vi "test-AprilTag-Test2.vi"() -> (3 "All Passed":bool)   [LabVIEW 2019]
uses:
  <vilib>/Rock Robotics/WPI/ThirdParty/JAS_Junk/TrajLib/TypeDef/AprilTagFieldLayout.ctl
  <vilib>/Rock Robotics/WPI/ThirdParty/JAS_Junk/TrajLib/TypeDef/AprilTag.ctl
  <vilib>/Rock Robotics/WPI/ThirdParty/JAS_Junk/TrajLib/TypeDef/POSE3D.ctl
  <vilib>/Rock Robotics/WPI/ThirdParty/JAS_Junk/TrajLib/TypeDef/TRANSLATION3D.ctl
  <vilib>/Rock Robotics/WPI/ThirdParty/JAS_Junk/TrajLib/TypeDef/ROTATION3D.ctl
  <vilib>/Rock Robotics/WPI/ThirdParty/JAS_Junk/TrajLib/TypeDef/QUATERNION.ctl
  <vilib>/Rock Robotics/WPI/ThirdParty/JAS_Junk/TrajLib/Enum/AprilTagFieldLayoutOrignPosition_ENUM.ctl
  <vilib>/Rock Robotics/WPI/ThirdParty/JAS_Junk/TrajLib/Conv_Deg_Radians.vi
  <vilib>/Rock Robotics/WPI/ThirdParty/JAS_Junk/TrajLib/VI/Quaternion_New.vi
  <vilib>/Rock Robotics/WPI/ThirdParty/JAS_Junk/TrajLib/VI/Translation3d_Create.vi
  <vilib>/Rock Robotics/WPI/ThirdParty/JAS_Junk/TrajLib/VI/Pose3d_New_Trans3dRot3d.vi
  <vilib>/Rock Robotics/WPI/ThirdParty/JAS_Junk/TrajLib/VI/AprilTag_GetAll.vi
  <vilib>/Rock Robotics/WPI/ThirdParty/JAS_Junk/TrajLib/VI/Pose3d_New_Default.vi
  <vilib>/Rock Robotics/WPI/ThirdParty/JAS_Junk/TrajLib/VI/Pose3d_RelativeTo.vi
  <vilib>/Rock Robotics/WPI/ThirdParty/JAS_Junk/TrajLib/VI/Translation3d_Equals.vi
  <vilib>/Rock Robotics/WPI/ThirdParty/JAS_Junk/TrajLib/VI/Rotation3d_Equals.vi
  <vilib>/Rock Robotics/WPI/ThirdParty/JAS_Junk/TrajLib/VI/Pose3d_getTranslation3d.vi
  <vilib>/Rock Robotics/WPI/ThirdParty/JAS_Junk/TrajLib/VI/Pose3d_getRotation3d.vi
  <vilib>/Rock Robotics/WPI/ThirdParty/JAS_Junk/TrajLib/VI/Translation3d_Create_Default.vi
  <vilib>/Rock Robotics/WPI/ThirdParty/JAS_Junk/TrajLib/VI/Rotation3d_Create_Default.vi
  <vilib>/Rock Robotics/WPI/ThirdParty/JAS_Junk/TrajLib/VI/Transform3d_Create_Pose3dPose3d.vi
  <vilib>/Rock Robotics/WPI/ThirdParty/JAS_Junk/TrajLib/VI/Transform3d_GetRotation3d.vi
  <vilib>/Rock Robotics/WPI/ThirdParty/JAS_Junk/TrajLib/VI/Transform3d_GetTranslation3d.vi
  <vilib>/Rock Robotics/WPI/ThirdParty/JAS_Junk/TrajLib/VI/Rotation3d_GetQuaterion.vi
  <vilib>/Rock Robotics/WPI/ThirdParty/JAS_Junk/TrajLib/VI/Quaternion_Equals.vi
  <vilib>/Rock Robotics/WPI/ThirdParty/JAS_Junk/TrajLib/VI/Quaternion_New_Default.vi
  <vilib>/Rock Robotics/WPI/ThirdParty/JAS_Junk/TrajLib/VI/Transform3d_Create_Trans3dRot3d.vi
  <vilib>/Rock Robotics/WPI/ThirdParty/JAS_Junk/TrajLib/VI/Translation3d_Minus.vi
  <vilib>/Rock Robotics/WPI/ThirdParty/JAS_Junk/TrajLib/VI/Translation3d_RotateBy.vi
  <vilib>/Rock Robotics/WPI/ThirdParty/JAS_Junk/TrajLib/VI/Rotation3d_UnaryMinus.vi
  <vilib>/Rock Robotics/WPI/ThirdParty/JAS_Junk/TrajLib/VI/Rotation3d_Minus.vi
  <vilib>/Rock Robotics/WPI/ThirdParty/JAS_Junk/TrajLib/VI/Quaternion_Get_Vect.vi
  <vilib>/Rock Robotics/WPI/ThirdParty/JAS_Junk/TrajLib/VI/Quaternion_Get_W.vi
  <vilib>/Rock Robotics/WPI/ThirdParty/JAS_Junk/TrajLib/VI/Quaternion_Times.vi
  <vilib>/Rock Robotics/WPI/ThirdParty/JAS_Junk/TrajLib/VI/Quaternion_Inverse.vi
  <vilib>/Rock Robotics/WPI/ThirdParty/JAS_Junk/TrajLib/VI/Quaternion_Get_All.vi
  <vilib>/Rock Robotics/WPI/ThirdParty/JAS_Junk/TrajLib/VI/Rotation3d_Create_Quaternion.vi
  <vilib>/Rock Robotics/WPI/ThirdParty/JAS_Junk/TrajLib/VI/Rotation3d_RotateBy.vi
  <vilib>/Rock Robotics/WPI/ThirdParty/JAS_Junk/TrajLib/VI/Quaternion_Normalize.vi
  <vilib>/Rock Robotics/WPI/ThirdParty/JAS_Junk/TrajLib/Trajectory_Library.lvlib
panel:
  out "Test 2 Passed":bool
  out "OriginPose3d":T1={"Translation3d"={"X"=0.0, "Y"=0.0, "Z"=0.0}, "Rotation3d"={"Q_quaternion"={"R"=1.0, "V"=[0.0, 0.0, 0.0]}}} {"Translation3d"."Z" format="%14.3f"; "Translation3d"."Y" format="%14.3f"; "Translation3d"."X" format="%14.3f"}
  out "AprilTagFieldLayout":T5={"AprilTagMap"={}, "FieldLength"=0.0, "FieldWidth"=0.0, "OriginPosition "=enum."kBlueAllianceWallRightSide,", "OriginPose3d"={"Translation3d"={"X"=0.0, "Y"=0.0, "Z"=0.0}, "Rotation3d"={"Q_quaternion"={"R"=1.0, "V"=[0.0, 0.0, 0.0]}}}} {"OriginPose3d"."Translation3d"."Z" format="%14.3f"; "OriginPose3d"."Translation3d"."Y" format="%14.3f"; "OriginPose3d"."Translation3d"."X" format="%14.3f"}
  out "Test 1 Passed":bool
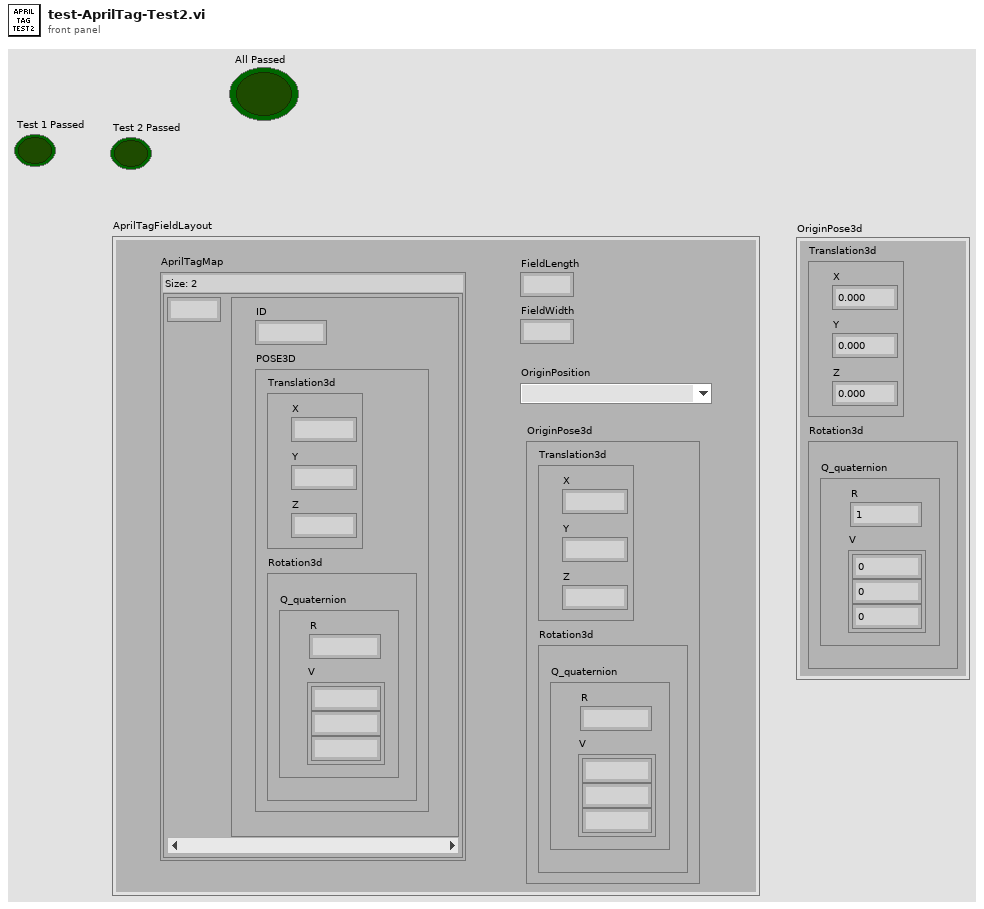
[diagram p1: front panel]
types:
  T1 = typedef "Trajectory_Library.lvlib/POSE3D.ctl" = cluster{"Translation3d":T2, "Rotation3d":T3}
  T2 = typedef "Trajectory_Library.lvlib/TRANSLATION3D.ctl" = cluster{"X":dbl, "Y":dbl, "Z":dbl}
  T3 = typedef "Trajectory_Library.lvlib/ROTATION3D.ctl" = cluster{"Q_quaternion":T4}
  T4 = typedef "Trajectory_Library.lvlib/QUATERNION.ctl" = cluster{"R":dbl, "V":dbl[]}
  T5 = typedef "Trajectory_Library.lvlib/AprilTagFieldLayout.ctl" = cluster{"AprilTagMap":map{i32, T6}, "FieldLength":dbl, "FieldWidth":dbl, "OriginPosition ":T7, "OriginPose3d":T1}
  T6 = typedef "Trajectory_Library.lvlib/AprilTag.ctl" = cluster{"ID":i32, "POSE3D":T1}
  T7 = typedef "Trajectory_Library.lvlib/AprilTagFieldLayoutOrignPosition_ENUM.ctl" = enum16{"kBlueAllianceWallRightSide,", "kRedAllianceWallRightSide,"}
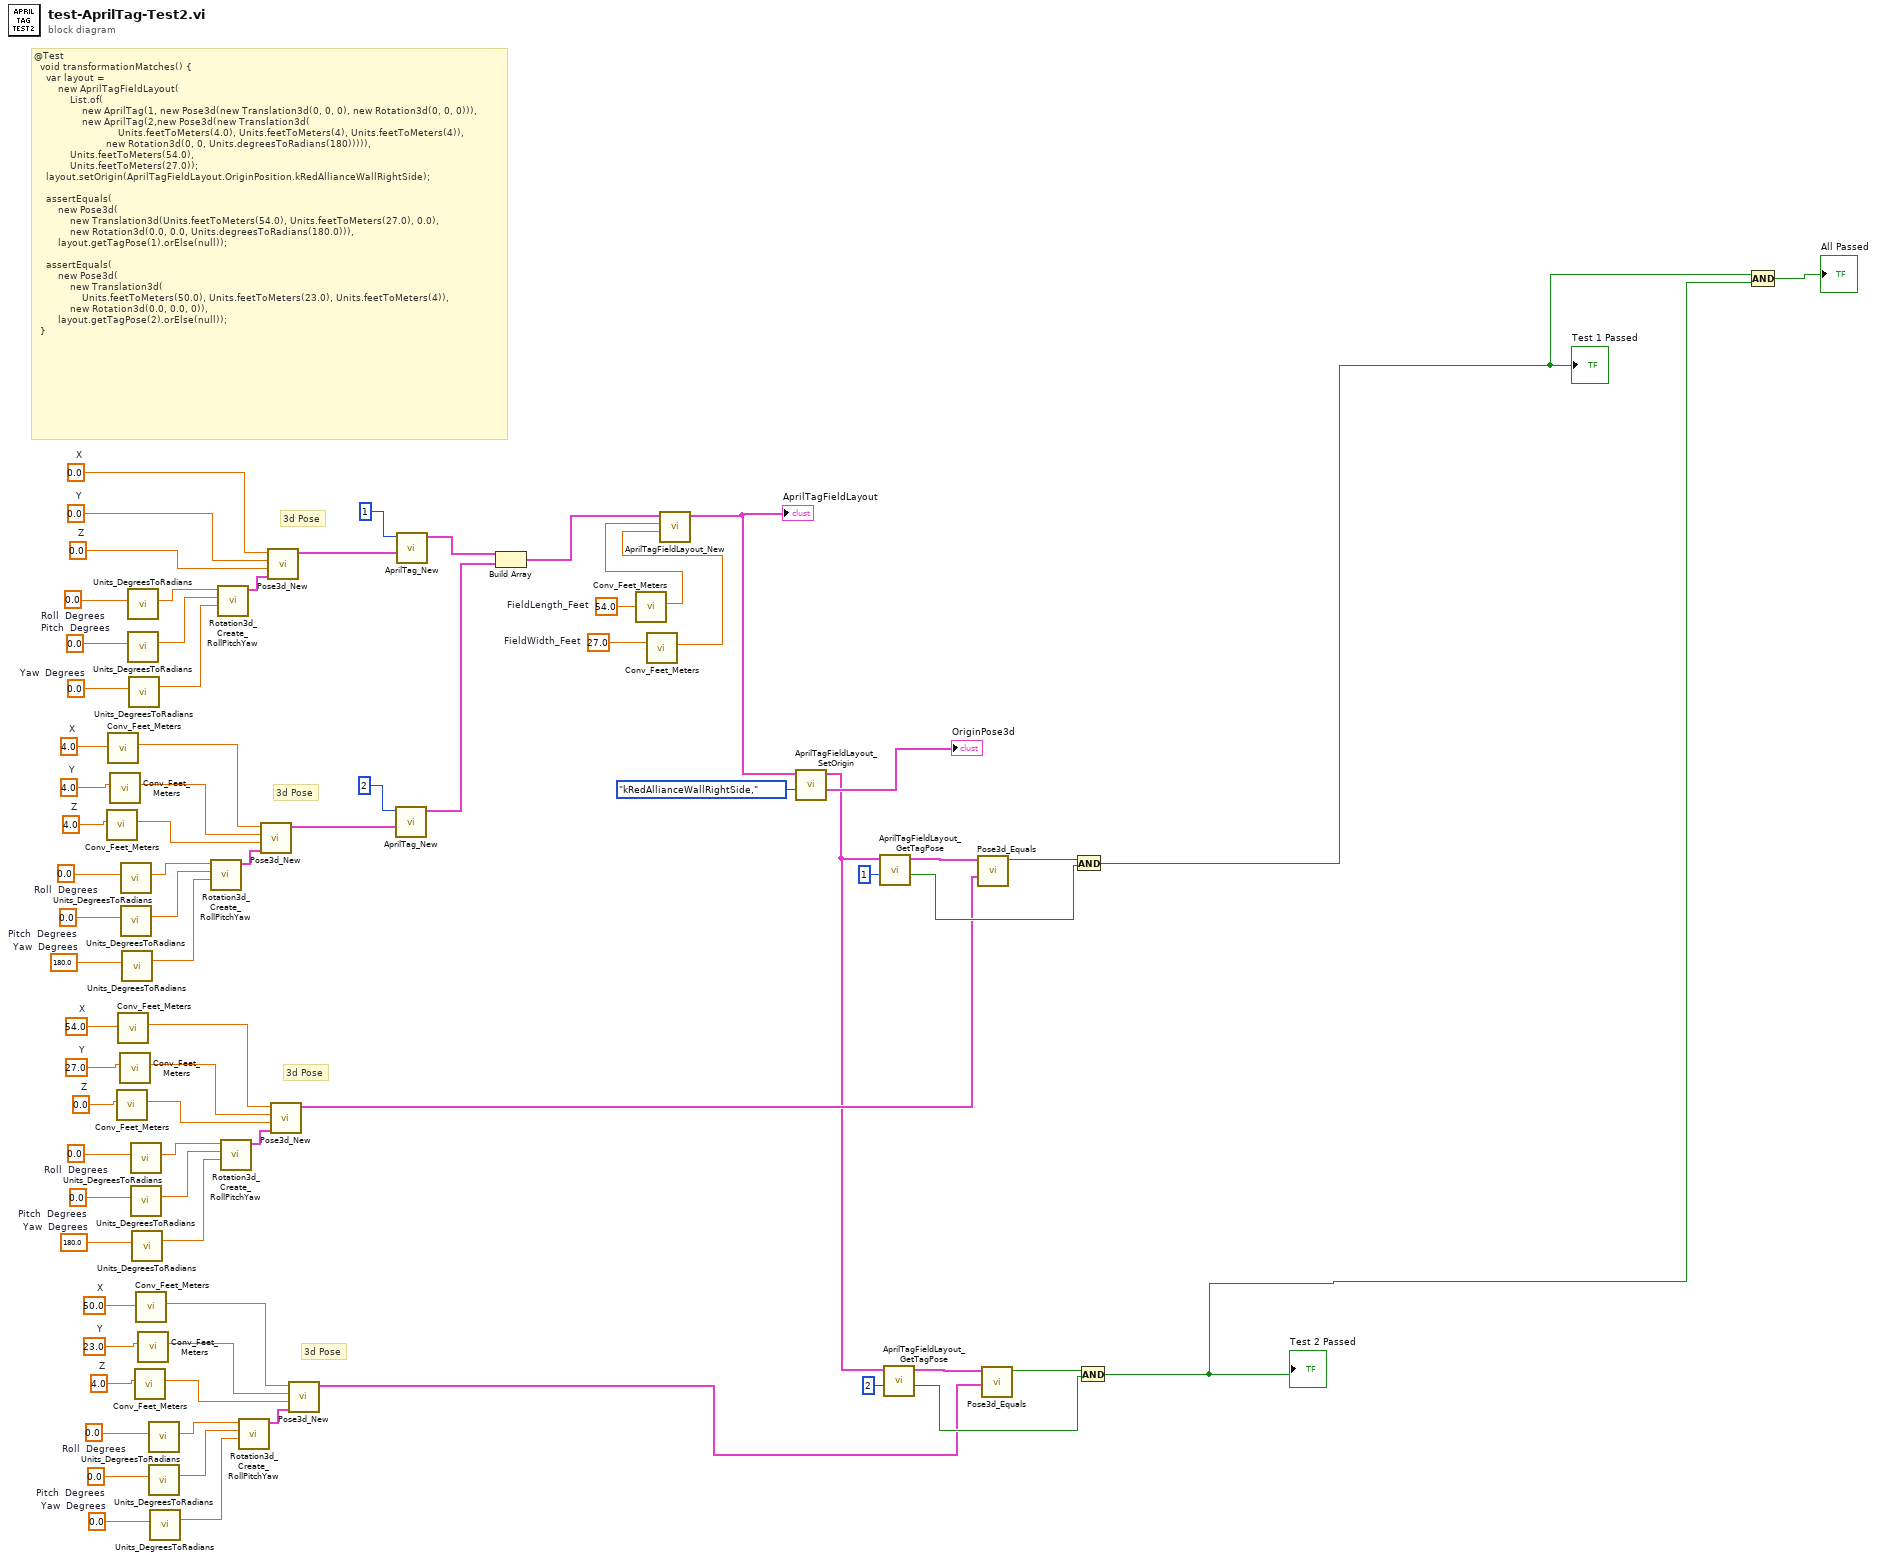
[diagram p0: block diagram]
diagram:
  w19 = 50.0  # X
  w20 = 23.0  # Y
  w21 = 4.0  # Z
  w25 = 0.0  # Roll  Degrees
  w26 = 0.0  # Pitch  Degrees
  w27 = 0.0  # Yaw  Degrees
  w32 = 54.0  # X
  w33 = 27.0  # Y
  w34 = 0.0  # Z
  w38 = 0.0  # Roll  Degrees
  w39 = 0.0  # Pitch  Degrees
  w40 = 180.0  # Yaw  Degrees
  w9 = 54.0  # FieldLength_Feet
  w8 = 27.0  # FieldWidth_Feet
  w47 = 4.0  # X
  w48 = 4.0  # Y
  w49 = 4.0  # Z
  w60 = 0.0  # Roll  Degrees
  w61 = 0.0  # Pitch  Degrees
  w62 = 180.0  # Yaw  Degrees
  w75 = 0.0  # X
  w74 = 0.0  # Y
  w73 = 0.0  # Z
  w67 = 0.0  # Roll  Degrees
  w68 = 0.0  # Pitch  Degrees
  w69 = 0.0  # Yaw  Degrees
  # "3d Pose"
  # "3d Pose"
  # "@Test\n  void transformationMatches() {\n    var layout =\n        new AprilTagFieldLayout(\n            List.of(\n                new AprilTag(1, new Pose3d(new Translation3d(0, 0, 0), new Rotation3d(0, 0, 0))),\n                new AprilTag(2,new Pose3d(new Translation3d(\n                            Units.feetToMeters(4.0), Units.feetToMeters(4), Units.feetToMeters(4)),\n                        new Rotation3d(0, 0, Units.degreesToRadians(180))))),\n            Units.feetToMeters(54.0),\n            Units.feetToMeters(27.0));\n    layout.setOrigin(AprilTagFieldLayout.OriginPosition.kRedAllianceWallRightSide);\n\n    assertEquals(\n        new Pose3d(\n            new Translation3d(Units.feetToMeters(54.0), Units.feetToMeters(27.0), 0.0),\n            new Rotation3d(0.0, 0.0, Units.degreesToRadians(180.0))),\n        layout.getTagPose(1).orElse(null));\n\n    assertEquals(\n        new Pose3d(\n            new Translation3d(\n                Units.feetToMeters(50.0), Units.feetToMeters(23.0), Units.feetToMeters(4)),\n            new Rotation3d(0.0, 0.0, 0)),\n        layout.getTagPose(2).orElse(null));\n  }"
  # "3d Pose"
  # "3d Pose"
  n1 = call <vilib>:"Conv_Feet_Meters.vi"("Feet"=w49) -> ("Meters"=w50:dbl)  [unwired: 10 in]
  n2 = call <vilib>:"Conv_Feet_Meters.vi"("Feet"=w47) -> ("Meters"=w52:dbl)  [unwired: 10 in]
  n3 = call <vilib>:"Conv_Feet_Meters.vi"("Feet"=w48) -> ("Meters"=w51:dbl)  [unwired: 10 in]
  n4 = call <vilib>:"Conv_Feet_Meters.vi"("Feet"=w34) -> ("Meters"=w35:dbl)  [unwired: 10 in]
  n5 = call <vilib>:"Conv_Feet_Meters.vi"("Feet"=w32) -> ("Meters"=w37:dbl)  [unwired: 10 in]
  n6 = call <vilib>:"Conv_Feet_Meters.vi"("Feet"=w33) -> ("Meters"=w36:dbl)  [unwired: 10 in]
  n7 = call <vilib>:"Units_DegreesToRadians.vi"("Degrees"=w60) -> ("Radians"=w63:dbl)  [unwired: 10 in]
  n8 = call <vilib>:"Units_DegreesToRadians.vi"("Degrees"=w61) -> ("Radians"=w64:dbl)  [unwired: 10 in]
  n9 = call <vilib>:"Units_DegreesToRadians.vi"("Degrees"=w62) -> ("Radians"=w65:dbl)  [unwired: 10 in]
  n10 = call <vilib>:"Units_DegreesToRadians.vi"("Degrees"=w67) -> ("Radians"=w70:dbl)  [unwired: 10 in]
  n11 = call <vilib>:"Units_DegreesToRadians.vi"("Degrees"=w68) -> ("Radians"=w71:dbl)  [unwired: 10 in]
  n12 = call <vilib>:"Units_DegreesToRadians.vi"("Degrees"=w69) -> ("Radians"=w72:dbl)  [unwired: 10 in]
  n13 = call <vilib>:"Units_DegreesToRadians.vi"("Degrees"=w38) -> ("Radians"=w41:dbl)  [unwired: 10 in]
  n14 = call <vilib>:"Units_DegreesToRadians.vi"("Degrees"=w39) -> ("Radians"=w42:dbl)  [unwired: 10 in]
  n15 = call <vilib>:"Units_DegreesToRadians.vi"("Degrees"=w40) -> ("Radians"=w43:dbl)  [unwired: 10 in]
  n16 = call <vilib>:"Conv_Feet_Meters.vi"("Feet"=w21) -> ("Meters"=w22:dbl)  [unwired: 10 in]
  n17 = call <vilib>:"Conv_Feet_Meters.vi"("Feet"=w19) -> ("Meters"=w24:dbl)  [unwired: 10 in]
  n18 = call <vilib>:"Conv_Feet_Meters.vi"("Feet"=w20) -> ("Meters"=w23:dbl)  [unwired: 10 in]
  n19 = call <vilib>:"Units_DegreesToRadians.vi"("Degrees"=w25) -> ("Radians"=w28:dbl)  [unwired: 10 in]
  n20 = call <vilib>:"Units_DegreesToRadians.vi"("Degrees"=w26) -> ("Radians"=w29:dbl)  [unwired: 10 in]
  n21 = call <vilib>:"Units_DegreesToRadians.vi"("Degrees"=w27) -> ("Radians"=w30:dbl)  [unwired: 10 in]
  n22 = call <vilib>:"Rotation3d_Create_RollPitchYaw.vi"("Yaw"=w65, "Pitch"=w64, "Roll"=w63) -> ("Rotation3d"=w66:T3)  [unwired: 8 in]
  n23 = call <vilib>:"Rotation3d_Create_RollPitchYaw.vi"("Yaw"=w72, "Pitch"=w71, "Roll"=w70) -> ("Rotation3d"=w76:T3)  [unwired: 8 in]
  n24 = call <vilib>:"Rotation3d_Create_RollPitchYaw.vi"("Yaw"=w43, "Pitch"=w42, "Roll"=w41) -> ("Rotation3d"=w44:T3)  [unwired: 8 in]
  n25 = call <vilib>:"Rotation3d_Create_RollPitchYaw.vi"("Yaw"=w30, "Pitch"=w29, "Roll"=w28) -> ("Rotation3d"=w31:T3)  [unwired: 8 in]
  n26 = call <vilib>:"Pose3d_New.vi"("Rotation3d"=w66, "z"=w50, "Y"=w51, "X"=w52) -> ("out Pose3d"=w56:T1)  [unwired: 7 in]
  n27 = call <vilib>:"Pose3d_New.vi"("Rotation3d"=w76, "z"=w73, "Y"=w74, "X"=w75) -> ("out Pose3d"=w58:T1)  [unwired: 7 in]
  n28 = call <vilib>:"Pose3d_New.vi"("Rotation3d"=w44, "z"=w35, "Y"=w36, "X"=w37) -> ("out Pose3d"=w14:T1)  [unwired: 7 in]
  n29 = call <vilib>:"Pose3d_New.vi"("Rotation3d"=w31, "z"=w22, "Y"=w23, "X"=w24) -> ("out Pose3d"=w2:T1)  [unwired: 7 in]
  n30 = call <vilib>:"AprilTag_New.vi"("POSE3D"=w56, "ID"=2) -> ("AprilTag"=w54:T6)  [unwired: 9 in]
  n31 = call <vilib>:"AprilTag_New.vi"("POSE3D"=w58, "ID"=1) -> ("AprilTag"=w55:T6)  [unwired: 9 in]
  n32 = Build Array(w55, w54) -> (w53:T6[])
  n33 = call <vilib>:"Conv_Feet_Meters.vi"("Feet"=w9) -> ("Meters"=w10:dbl)  [unwired: 10 in]
  n34 = call <vilib>:"Conv_Feet_Meters.vi"("Feet"=w8) -> ("Meters"=w11:dbl)  [unwired: 10 in]
  n35 = call <vilib>:"AprilTagFieldLayout_New.vi"("FieldWidth_Meters"=w11, "FieldLength_Meters"=w10, "AprilTags"=w53) -> ("AprilTagFieldLayout"=w46:T5)  [unwired: 8 in]
  "AprilTagFieldLayout" <- w46
  n36 = call <vilib>:"AprilTagFieldLayout_SetOrigin.vi"("OriginPosition"=AprilTagFieldLayoutOrignPosition_ENUM."kRedAllianceWallRightSide,", "in AprilTagFieldLayout"=w46) -> ("OriginPose3d"=→"OriginPose3d":T1, "out AprilTagFieldLayout"=w3:T5)  [unwired: 8 in]
  n37 = call <vilib>:"AprilTagFieldLayout_GetTagPose.vi"("TagId"=1, "AprilTagFieldLayout"=w3) -> ("Found"=w15:bool, "TagPose3d"=w17:T1)  [unwired: 8 in]
  n38 = call <vilib>:"AprilTagFieldLayout_GetTagPose.vi"("TagId"=2, "AprilTagFieldLayout"=w3) -> ("Found"=w4:bool, "TagPose3d"=w6:T1)  [unwired: 8 in]
  n39 = call <vilib>:"Pose3d_Equals.vi"("other Pose3d"=w14, "in Pose3d"=w17) -> ("Equals"=w16:bool)  [unwired: 9 in]
  n40 = call <vilib>:"Pose3d_Equals.vi"("other Pose3d"=w2, "in Pose3d"=w6) -> ("Equals"=w5:bool)  [unwired: 9 in]
  n41 = And(x=w16, y=w15) -> (x .and. y?=w13:bool)
  "Test 1 Passed" <- w13
  n42 = And(x=w5, y=w4) -> (x .and. y?=w1:bool)
  "Test 2 Passed" <- w1
  n43 = Compound Arithmetic op=AND(w13, w1) -> (→"All Passed":bool)
